vi "Read E-Series File Names.vi"(8 "error in (no error)":errorcluster, 11 "INI File":string="e-series files names.ini") -> (0 "error out":errorcluster, 3 "E-Series File Names":string[](array[string]))   [LabVIEW 2018]
uses:
  <vilib>/Utility/config.llb/Read Key (String).vi
  <vilib>/Utility/config.llb/NI_LVConfig.lvlib
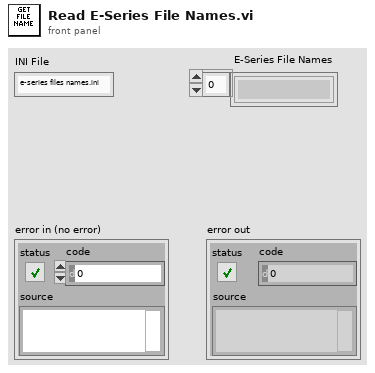
[diagram p1: front panel]
types:
  T1 = typedef "NI_LVConfig.lvlib/Config Data RefNum.ctl" = refnum<k1>
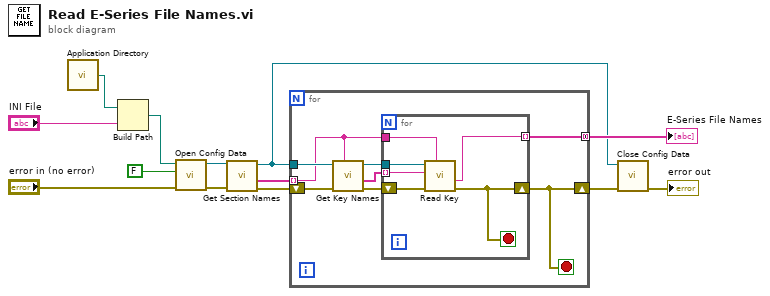
[diagram p0: block diagram]
diagram:
  n1 = call <vilib>:"Application Directory.vi"() -> ("Application Directory"=w12:path)
  n2 = Build Path(base path=w12, name or relative path="INI File") -> (appended path=w11:path)
  n3 = call <vilib>:"Open Config Data.vi"("error in (no error)"="error in (no error)", "create file if necessary (T)"=FALSE, "configuration file path"=w11) -> ("error out"=w8:errorcluster, "refnum"=w9:T1)  [unwired: 6 in, 1 out]
  n4 = call <vilib>:"Get Section Names.vi"("error in (no error)"=w8, "refnum"=w9) -> ("error out"=w7:errorcluster, "section names"=w6:string[], "refnum out"=w1:T1)  [unwired: 7 in]
  n5 = for {
    shift-right: [w17] -> w3
    shift-left: w7 -> [w21]
    tunnel: w1 -> [w20]
    tunnel: w6 -> [w16] mode=indexing
    tunnel: [w15] -> w4 mode=concatenating
    stop <- w17 stop-if-true
    n6 = call <vilib>:"Get Key Names.vi"("section"=w16, "error in (no error)"=w21, "refnum"=w20) -> ("error out"=w19:errorcluster, "key names"=w14:string[], "refnum out"=w18:T1)  [unwired: 5 in, 1 out]
    n7 = for {
      shift-right: [w25] -> w17
      shift-left: w19 -> [w27]
      tunnel: w16 -> [w24]
      tunnel: w18 -> [w26]
      tunnel: [w23] -> w15 mode=indexing
      tunnel: w14 -> [w22] mode=indexing
      stop <- w25 stop-if-true
      n8 = call-poly <vilib>:"Read Key.vi"("section"=w24, "error in (no error)"=w27, "key"=w22, "refnum"=w26) -> ("error out"=w25:errorcluster, "value"=w23:string)  [unwired: 4 in, 2 out]
    }
  }
  "E-Series File Names" <- w4
  n9 = call <vilib>:"Close Config Data.vi"("error in (no error)"=w3, "refnum"=w1) -> ("error out"=→"error out":errorcluster)  [unwired: 8 in, 1 out]
